vi "1599 UI.vi"() -> ()   [LabVIEW 2015]
uses:
  <vilib>/LabVIEW Interface for Arduino/Type Defs/Pin Mode.ctl
  <vilib>/LabVIEW Interface for Arduino/Type Defs/Board Type.ctl
  C:/Users/adahal/Desktop/AJ/Projects/LABVIEW/1599/From Zach/QuickLaserFactoryCalibration.dll
  From Zach/QuickLaserFactoryCalibration.dll
  <vilib>/LabVIEW Interface for Arduino/LabVIEW Interface for Arduino.lvlib
panel:
  out "Tab Control":T1(tab)
  in  "InitializeTest":bool
  in  "stop":bool
  out "String":string
  in  "Page 2 continue":bool
  out "Page 2 continue":string
  in  "Start Test":bool
  out "Progress Bar":u8(slide) scale=0.0..100.0
  out "String 5":string
  in  "stop Error":bool
  in  "Finish":bool
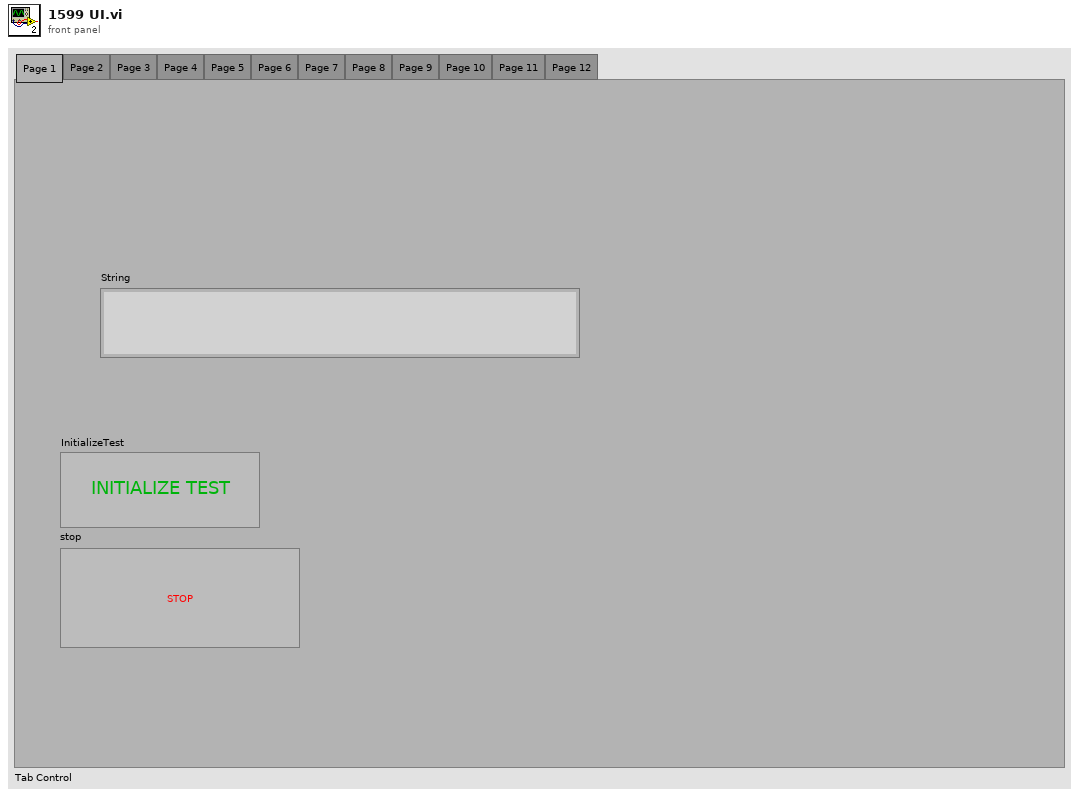
[diagram p1: front panel]
types:
  T1 = enum32{"Page 1", "Page 2", "Page 3", "Page 4", "Page 5", "Page 6", "Page 7", "Page 8", "Page 9", "Page 10", "Page 11", "Page 12"}
  T2 = typedef "LabVIEW Interface for Arduino.lvlib/Board Type.ctl" = enum16{"Uno", "Dimuelanove w/Atmega 328", "Mega 2560"}
  T3 = typedef "LabVIEW Interface for Arduino.lvlib/Pin Mode.ctl" = enum8{"Input", "Output"}
  T4 = enum32{"Page 1", "Page 2", "Page 3", "Page 4", "Page 5"}
  T5 = typedef "LabVIEW Interface for Arduino.lvlib/Arduino Resource.ctl" = cluster{"VISA resource":refnum<visa-resource-name>, "Board Type":T2, "Connection Type":enum8{"USB / Serial"}, "Bytes Per Packet (15)":u8}
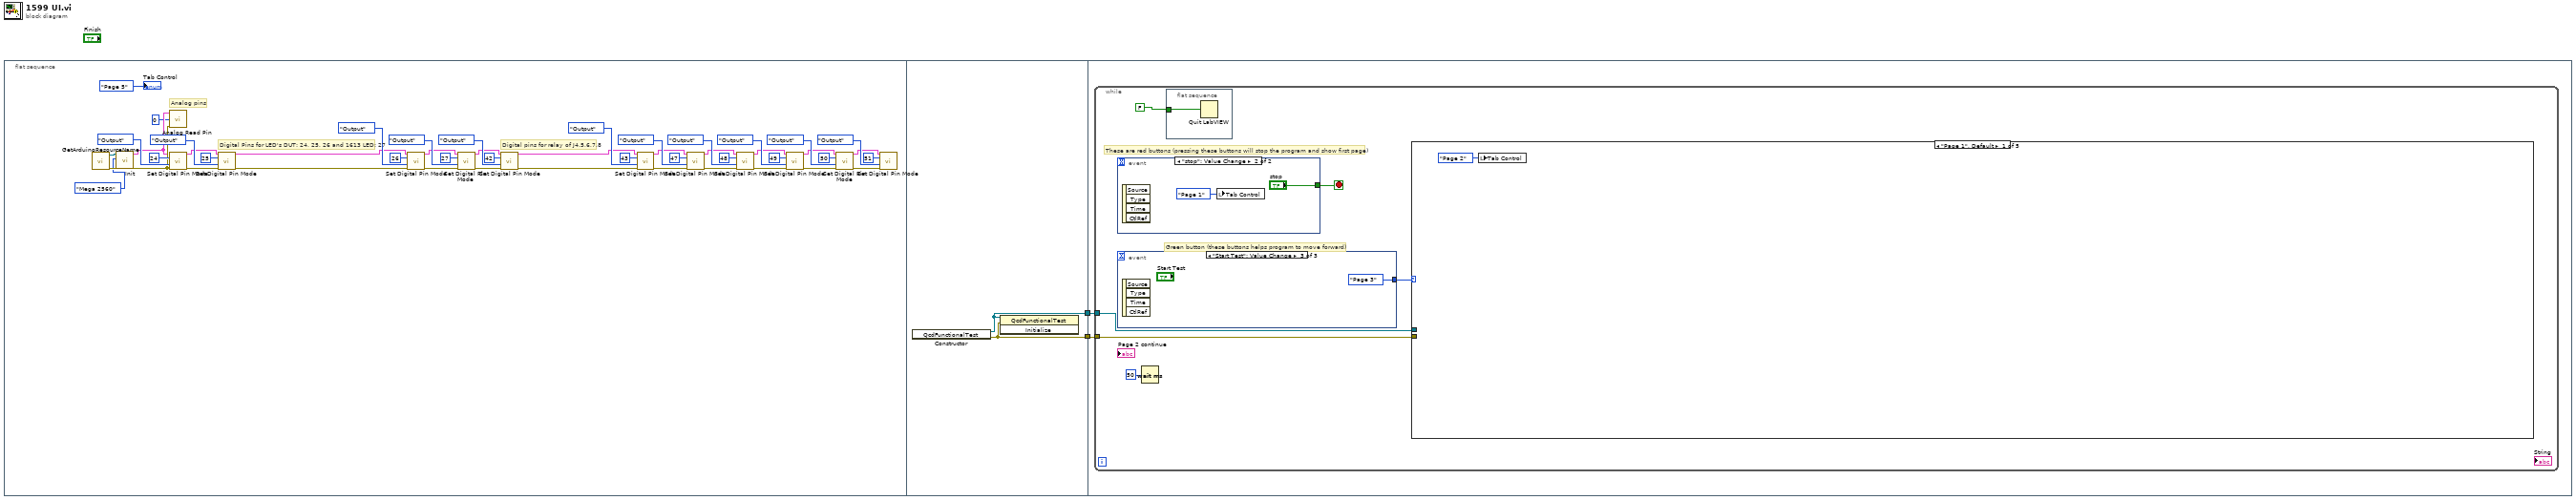
[diagram p0: block diagram]
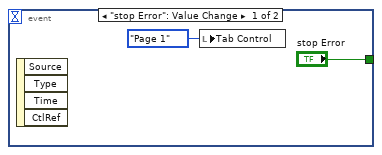
[diagram p2: hidden frame]
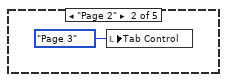
[diagram p3: hidden frame]
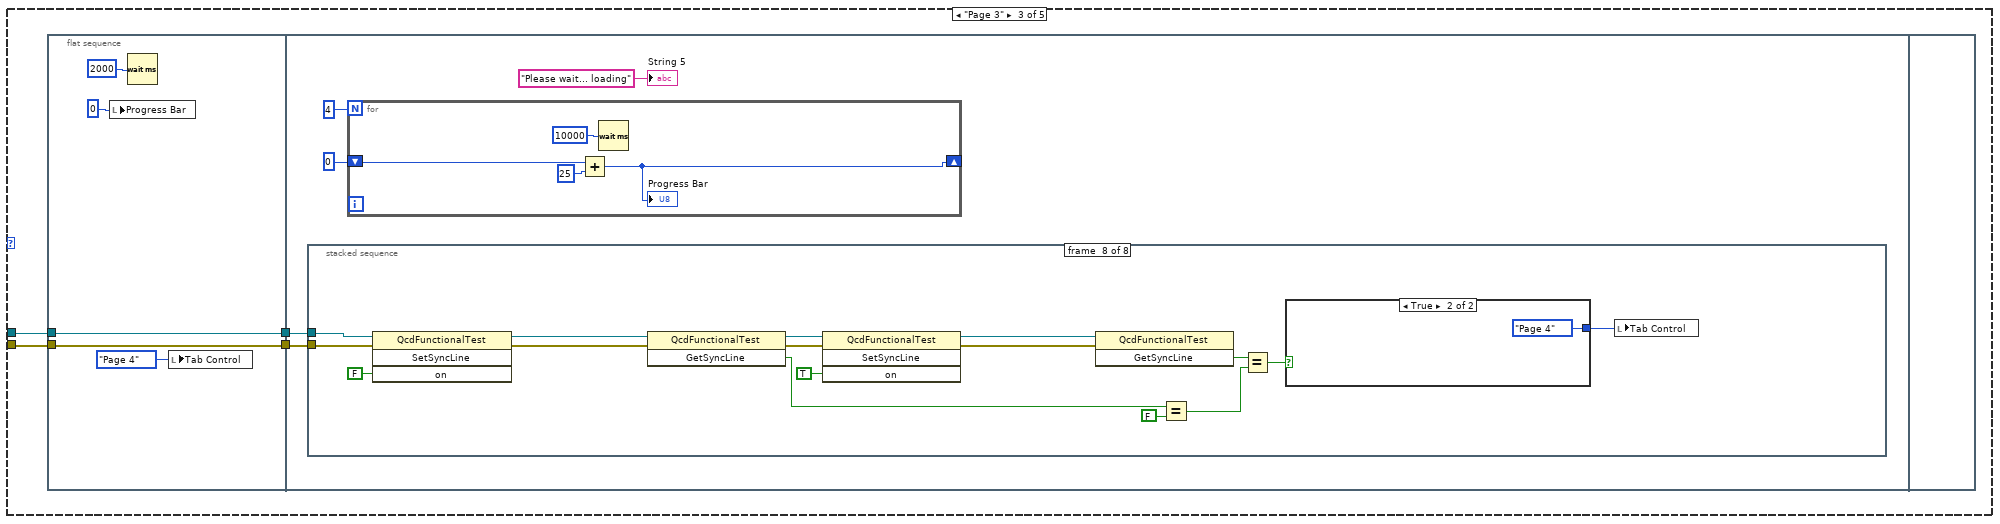
[diagram p4: hidden frame]
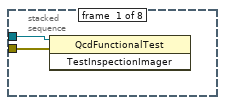
[diagram p5: hidden frame]
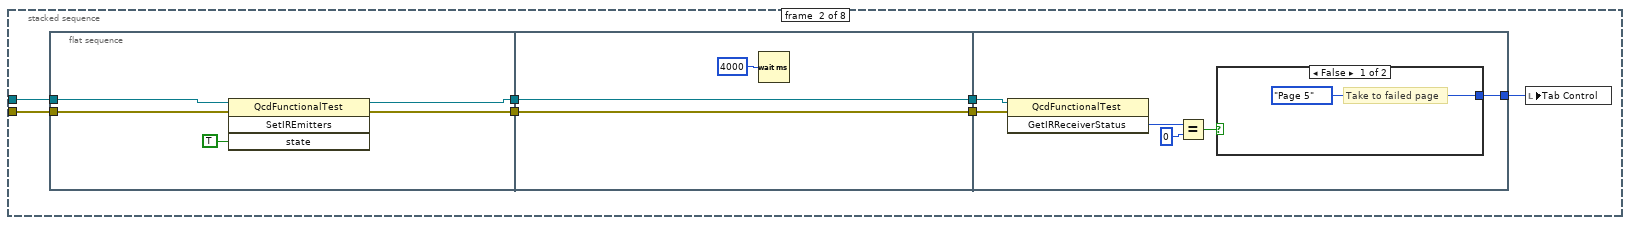
[diagram p6: hidden frame]
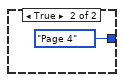
[diagram p7: hidden frame]
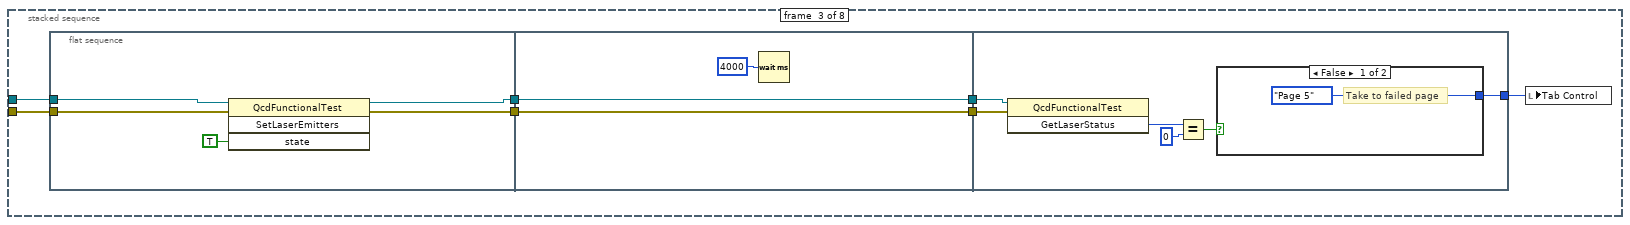
[diagram p8: hidden frame]
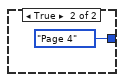
[diagram p9: hidden frame]
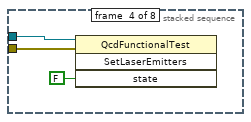
[diagram p10: hidden frame]
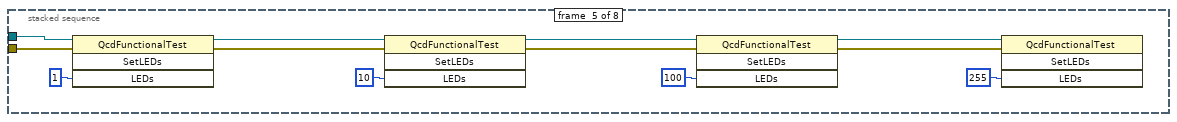
[diagram p11: hidden frame]
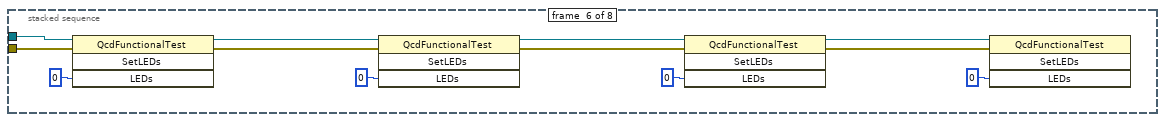
[diagram p12: hidden frame]
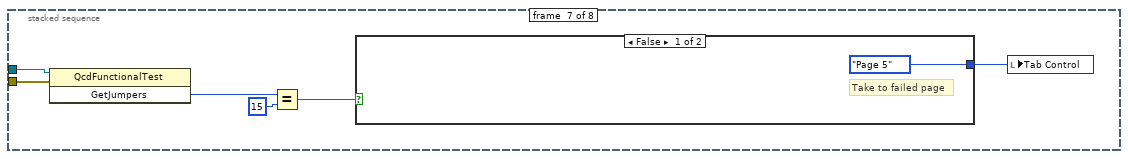
[diagram p13: hidden frame]
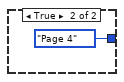
[diagram p14: hidden frame]
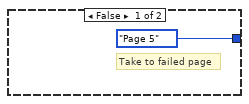
[diagram p15: hidden frame]
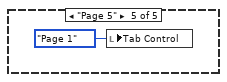
[diagram p17: hidden frame]
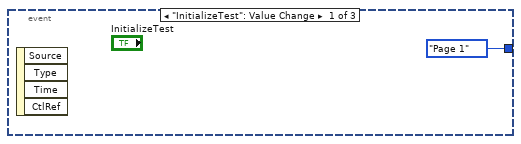
[diagram p18: hidden frame]
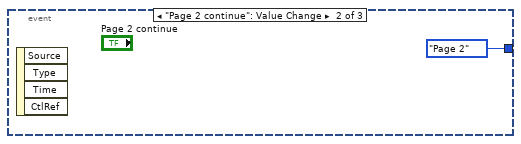
[diagram p19: hidden frame]
diagram:
  n1 = flat-sequence {
    tunnel: [w53] -> w2
    tunnel: [w52] -> w1
    tunnel: w2 -> [w55]
    tunnel: w1 -> [w54]
    frame #0 {
      # "Digital pins for relay of J4,5,6,7,8"
      # "Digital Pins for LED's DUT: 24, 25, 26 and 1613 LED: 27"
      # "Analog pins"
      n2 = call "GetArduinoResourceName.vi"() -> ("error out"=w5:errorcluster, "VISA resource name"=w6:refnum<visa-resource-name>)  [unwired: 10 in]
      n3 = call <vilib>:"Init.vi"("VISA resource"=w6, "Board Type (Uno)"=Board_Type."Mega 2560", "error in"=w5) -> ("Arduino Resource"=w17:T5, "error out"=w18:errorcluster)  [unwired: 15 in]
      n4 = call <vilib>:"Analog Read Pin.vi"("Arduino Resource"=w17, "Analog Input Pin (0)"=u8 0, "error in"=w18) -> ()  [unwired: 10 in, 3 out]
      n5 = call <vilib>:"Set Digital Pin Mode.vi"("Arduino Resource"=w17, "Digital I/O Pin"=u8 24, "Pin Mode (Input)"=Pin_Mode."Output", "error in"=w18) -> ("Arduino Resource"=w7:T5, "error out"=w8:errorcluster)  [unwired: 10 in]
      n6 = call <vilib>:"Set Digital Pin Mode.vi"("Arduino Resource"=w7, "Digital I/O Pin"=u8 25, "Pin Mode (Input)"=Pin_Mode."Output", "error in"=w8) -> ("Arduino Resource"=w9:T5, "error out"=w10:errorcluster)  [unwired: 10 in]
      n7 = call <vilib>:"Set Digital Pin Mode.vi"("Arduino Resource"=w9, "Digital I/O Pin"=u8 26, "Pin Mode (Input)"=Pin_Mode."Output", "error in"=w10) -> ("Arduino Resource"=w11:T5, "error out"=w12:errorcluster)  [unwired: 10 in]
      n8 = call <vilib>:"Set Digital Pin Mode.vi"("Arduino Resource"=w11, "Digital I/O Pin"=u8 27, "Pin Mode (Input)"=Pin_Mode."Output", "error in"=w12) -> ("Arduino Resource"=w13:T5, "error out"=w14:errorcluster)  [unwired: 10 in]
      n9 = call <vilib>:"Set Digital Pin Mode.vi"("Arduino Resource"=w13, "Digital I/O Pin"=u8 42, "Pin Mode (Input)"=Pin_Mode."Output", "error in"=w14) -> ("Arduino Resource"=w15:T5, "error out"=w16:errorcluster)  [unwired: 10 in]
      n10 = call <vilib>:"Set Digital Pin Mode.vi"("Arduino Resource"=w15, "Digital I/O Pin"=u8 43, "Pin Mode (Input)"=Pin_Mode."Output", "error in"=w16) -> ("Arduino Resource"=w31:T5, "error out"=w32:errorcluster)  [unwired: 10 in]
      n11 = call <vilib>:"Set Digital Pin Mode.vi"("Arduino Resource"=w31, "Digital I/O Pin"=u8 47, "Pin Mode (Input)"=Pin_Mode."Output", "error in"=w32) -> ("Arduino Resource"=w33:T5, "error out"=w34:errorcluster)  [unwired: 10 in]
      n12 = call <vilib>:"Set Digital Pin Mode.vi"("Arduino Resource"=w33, "Digital I/O Pin"=u8 48, "Pin Mode (Input)"=Pin_Mode."Output", "error in"=w34) -> ("Arduino Resource"=w35:T5, "error out"=w36:errorcluster)  [unwired: 10 in]
      n13 = call <vilib>:"Set Digital Pin Mode.vi"("Arduino Resource"=w35, "Digital I/O Pin"=u8 49, "Pin Mode (Input)"=Pin_Mode."Output", "error in"=w36) -> ("Arduino Resource"=w37:T5, "error out"=w38:errorcluster)  [unwired: 10 in]
      n14 = call <vilib>:"Set Digital Pin Mode.vi"("Arduino Resource"=w37, "Digital I/O Pin"=u8 50, "Pin Mode (Input)"=Pin_Mode."Output", "error in"=w38) -> ("Arduino Resource"=w39:T5, "error out"=w40:errorcluster)  [unwired: 10 in]
      n15 = call <vilib>:"Set Digital Pin Mode.vi"("Arduino Resource"=w39, "Digital I/O Pin"=u8 51, "Pin Mode (Input)"=Pin_Mode."Output", "error in"=w40) -> ()  [unwired: 10 in, 2 out]
      "Tab Control" <- T4."Page 5" ("Tab Control")
    }
    frame #1 {
      n16 = constructor class="QcdFunctionalTest"() -> (reference out=w53:refnum<k24>, error out=w52:errorcluster)  [unwired: 3 in, 1 out]
      n17 = invoke class="QcdFunctionalTest" method="Initialize"(reference=w53, error in=w52) -> ()  [unwired: 1 in, 3 out]
    }
    frame #2 {
      n18 = while {
        tunnel: w55 -> [w58]
        tunnel: w54 -> [w57]
        stop <- w56 stop-if-true
        # "These are red buttons (pressing these buttons will stop the program and show first page)"
        # "Green button (these buttons helps program to move forward)"
        n19 = event shown="[1] \"stop\": Value Change" {
          selector: _ -> [_ _]
          dyn-events: _ -> [_ _]
          timeout: _ -> [_ _]
          tunnel: ["stop Error" "stop"] -> w56
          event "stop Error": Value Change {
            n20 = event-data() -> ()  [unwired: 1 in, 4 out]
            n21 = local write "Tab Control"(T1."Page 1" ("Tab Control")) -> ()
          }
          event "stop": Value Change {
            n22 = event-data() -> ()  [unwired: 1 in, 4 out]
            n23 = local write "Tab Control"(T1."Page 1" ("Tab Control")) -> ()
          }
        }
        n24 = event shown="[2] \"Start Test\": Value Change" {
          selector: _ -> [_ _ _]
          dyn-events: _ -> [_ _ _]
          timeout: _ -> [_ _ _]
          tunnel: [enum32{"Page 1", "Page 2"}."Page 1" ("Tab Control") enum32{"Page 1", "Page 2"}."Page 2" ("Tab Control") T4."Page 3" ("Tab Control")] -> w61
          event "InitializeTest": Value Change {
            n25 = event-data() -> ()  [unwired: 1 in, 4 out]
          }
          event "Page 2 continue": Value Change {
            n26 = event-data() -> ()  [unwired: 1 in, 4 out]
          }
          event "Start Test": Value Change {
            n27 = event-data() -> ()  [unwired: 1 in, 4 out]
          }
        }
        n28 = Wait (ms)(milliseconds to wait=u32 50) -> ()  [unwired: 1 out]
        n29 = flat-sequence {
          tunnel: FALSE -> [w66]
          frame #0 {
            n30 = Quit LabVIEW(quit? (T)=w66) -> ()
          }
        }
        n31 = case shown="\"Page 1\", Default" w61 {
          tunnel: w58 -> [_ _ w71 _ _]
          tunnel: w57 -> [_ _ w69 _ _]
          frame "Page 1", Default {
            n32 = local write "Tab Control"(enum32{"Page 1", "Page 2"}."Page 2" ("Tab Control")) -> ()
          }
          frame "Page 2" {
            n33 = local write "Tab Control"(T4."Page 3" ("Tab Control")) -> ()
          }
          frame "Page 3" {
            n34 = flat-sequence {
              tunnel: [w74] -> w72
              tunnel: w71 -> [w74]
              tunnel: [w73] -> w70
              tunnel: w69 -> [w73]
              tunnel: w72 -> [w79]
              tunnel: w70 -> [w78]
              frame #0 {
                n35 = local write "Progress Bar"(u8 0 ("Progress Bar")) -> ()
                n36 = Wait (ms)(milliseconds to wait=u32 2000) -> ()  [unwired: 1 out]
                n37 = local write "Tab Control"(T4."Page 4" ("Tab Control")) -> ()
              }
              frame #1 {
                n38 = stacked-sequence {
                  tunnel: w78 -> [w83 w90 w113 w132 w144 w146 w162 w167]
                  tunnel: w79 -> [w84 w91 w114 w133 w145 w147 w163 w166]
                  frame #0 {
                    n39 = invoke class="QcdFunctionalTest" method="TestInspectionImager"(reference=w84, error in=w83) -> ()  [unwired: 1 in, 3 out]
                  }
                  frame #1 {
                    n40 = flat-sequence {
                      tunnel: w91 -> [w95]
                      tunnel: w90 -> [w94]
                      tunnel: [w93] -> w88
                      tunnel: [w92] -> w86
                      tunnel: [w99] -> w89
                      tunnel: w88 -> [w99]
                      tunnel: [w98] -> w87
                      tunnel: w86 -> [w98]
                      tunnel: w89 -> [w105]
                      tunnel: w87 -> [w104]
                      tunnel: [w100] -> w85
                      frame #0 {
                        n41 = invoke class="QcdFunctionalTest" method="SetIREmitters"(reference=w95, error in=w94, "state"=TRUE) -> (reference out=w93:refnum<k24>, error out=w92:errorcluster)  [unwired: 1 in, 2 out]
                      }
                      frame #1 {
                        n42 = Wait (ms)(milliseconds to wait=u32 4000) -> ()  [unwired: 1 out]
                      }
                      frame #2 {
                        n43 = invoke class="QcdFunctionalTest" method="GetIRReceiverStatus"(reference=w105, error in=w104) -> ("GetIRReceiverStatus"=w103:u8)  [unwired: 1 in, 2 out]
                        n44 = Equal?(x=w103, y=u8 0 ("GetIRReceiverStatus")) -> (x = y?=w101:bool)
                        n45 = case shown="False" w101 {
                          tunnel: [T4."Page 5" ("Tab Control") T4."Page 4" ("Tab Control")] -> w100
                          frame False {
                            # "Take to failed page"
                          }
                          frame True {
                          }
                        }
                      }
                    }
                    n46 = local write "Tab Control"(w85) -> ()
                  }
                  frame #2 {
                    n47 = flat-sequence {
                      tunnel: w114 -> [w119]
                      tunnel: w113 -> [w118]
                      tunnel: [w116] -> w111
                      tunnel: [w115] -> w109
                      tunnel: [w121] -> w112
                      tunnel: w111 -> [w121]
                      tunnel: [w120] -> w110
                      tunnel: w109 -> [w120]
                      tunnel: w112 -> [w127]
                      tunnel: w110 -> [w128]
                      tunnel: [w123] -> w108
                      frame #0 {
                        n48 = invoke class="QcdFunctionalTest" method="SetLaserEmitters"(reference=w119, error in=w118, "state"=TRUE) -> (reference out=w115:refnum<k24>, error out=w116:errorcluster)  [unwired: 1 in, 2 out]
                      }
                      frame #1 {
                        n49 = Wait (ms)(milliseconds to wait=u32 4000) -> ()  [unwired: 1 out]
                      }
                      frame #2 {
                        n50 = invoke class="QcdFunctionalTest" method="GetLaserStatus"(reference=w128, error in=w127) -> ("GetLaserStatus"=w126:u8)  [unwired: 1 in, 2 out]
                        n51 = Equal?(x=w126, y=u8 0 ("GetLaserStatus")) -> (x = y?=w124:bool)
                        n52 = case shown="False" w124 {
                          tunnel: [T4."Page 5" ("Tab Control") T4."Page 4" ("Tab Control")] -> w123
                          frame False {
                            # "Take to failed page"
                          }
                          frame True {
                          }
                        }
                      }
                    }
                    n53 = local write "Tab Control"(w108) -> ()
                  }
                  frame #3 {
                    n54 = invoke class="QcdFunctionalTest" method="SetLaserEmitters"(reference=w133, error in=w132, "state"=FALSE) -> ()  [unwired: 1 in, 4 out]
                  }
                  frame #4 {
                    n55 = invoke class="QcdFunctionalTest" method="SetLEDs"(reference=w145, error in=w144, "LEDs"=u8 1) -> (reference out=w139:refnum<k24>, error out=w138:errorcluster)  [unwired: 1 in, 2 out]
                    n56 = invoke class="QcdFunctionalTest" method="SetLEDs"(reference=w139, error in=w138, "LEDs"=u8 10) -> (reference out=w136:refnum<k24>, error out=w137:errorcluster)  [unwired: 1 in, 2 out]
                    n57 = invoke class="QcdFunctionalTest" method="SetLEDs"(reference=w136, error in=w137, "LEDs"=u8 100) -> (reference out=w135:refnum<k24>, error out=w134:errorcluster)  [unwired: 1 in, 2 out]
                    n58 = invoke class="QcdFunctionalTest" method="SetLEDs"(reference=w135, error in=w134, "LEDs"=u8 255) -> ()  [unwired: 1 in, 4 out]
                  }
                  frame #5 {
                    n59 = invoke class="QcdFunctionalTest" method="SetLEDs"(reference=w147, error in=w146, "LEDs"=u8 0) -> (reference out=w149:refnum<k24>, error out=w150:errorcluster)  [unwired: 1 in, 2 out]
                    n60 = invoke class="QcdFunctionalTest" method="SetLEDs"(reference=w149, error in=w150, "LEDs"=u8 0) -> (reference out=w152:refnum<k24>, error out=w153:errorcluster)  [unwired: 1 in, 2 out]
                    n61 = invoke class="QcdFunctionalTest" method="SetLEDs"(reference=w152, error in=w153, "LEDs"=u8 0) -> (reference out=w154:refnum<k24>, error out=w155:errorcluster)  [unwired: 1 in, 2 out]
                    n62 = invoke class="QcdFunctionalTest" method="SetLEDs"(reference=w154, error in=w155, "LEDs"=u8 0) -> ()  [unwired: 1 in, 4 out]
                  }
                  frame #6 {
                    n63 = invoke class="QcdFunctionalTest" method="GetJumpers"(reference=w163, error in=w162) -> ("GetJumpers"=w161:u8)  [unwired: 1 in, 2 out]
                    n64 = Equal?(x=w161, y=u8 15 ("GetJumpers")) -> (x = y?=w159:bool)
                    n65 = case shown="False" w159 {
                      tunnel: [T4."Page 5" ("Tab Control") T4."Page 4" ("Tab Control")] -> w158
                      frame False {
                        # "Take to failed page"
                      }
                      frame True {
                      }
                    }
                    n66 = local write "Tab Control"(w158) -> ()
                  }
                  frame #7 {
                    n67 = invoke class="QcdFunctionalTest" method="SetSyncLine"(reference=w166, error in=w167, "on"=FALSE) -> (reference out=w180:refnum<k24>, error out=w179:errorcluster)  [unwired: 1 in, 2 out]
                    n68 = invoke class="QcdFunctionalTest" method="GetSyncLine"(reference=w180, error in=w179) -> (reference out=w176:refnum<k24>, error out=w175:errorcluster, "GetSyncLine"=w177:bool)  [unwired: 1 in]
                    n69 = invoke class="QcdFunctionalTest" method="SetSyncLine"(reference=w176, error in=w175, "on"=TRUE) -> (reference out=w173:refnum<k24>, error out=w172:errorcluster)  [unwired: 1 in, 2 out]
                    n70 = invoke class="QcdFunctionalTest" method="GetSyncLine"(reference=w173, error in=w172) -> ("GetSyncLine"=w171:bool)  [unwired: 1 in, 2 out]
                    n71 = Equal?(x=w177, y=FALSE ("on")) -> (x = y?=w170:bool)
                    n72 = Equal?(x=w171, y=w170) -> (x = y?=w169:bool)
                    n73 = case shown="True" w169 {
                      tunnel: [T4."Page 5" ("Tab Control") T4."Page 4" ("Tab Control")] -> w168
                      frame False {
                        # "Take to failed page"
                      }
                      frame True {
                      }
                    }
                    n74 = local write "Tab Control"(w168) -> ()
                  }
                }
                n75 = for {
                  N: 4 -> [_]
                  shift-right: [w185] -> _
                  shift-left: 0 -> [w184]
                  n76 = Add(x=w184, y=25) -> (x+y=w185:i32)
                  "Progress Bar" <- w185
                  n77 = Wait (ms)(milliseconds to wait=u32 10000) -> ()  [unwired: 1 out]
                }
                "String 5" <- "Please wait... loading" ("String 5")
              }
              frame #2 {
              }
            }
          }
          frame "Page 4" {
          }
          frame "Page 5" {
            n78 = local write "Tab Control"(T4."Page 1" ("Tab Control")) -> ()
          }
        }
      }
    }
  }
